vi "Handle Errors.vi"(8 "error in (no error)":errorcluster, 10 "Location":string, 11 "Mock Error Handler In":refnum<class "Mock Error Handler.lvclass">) -> (0 "error out":errorcluster, 3 "Mock Error Handler Out":refnum<class "Mock Error Handler.lvclass">)   [LabVIEW 2020, in "Mock Error Handler.lvclass"]
uses:
  Mock Error Handler.lvclass
  C:/Users/anton/Documents/GitHub/Triarc-Framework/source/Framework/Process/Process.lvclass
  Private/Error Message Data.ctl
  Framework/Process/Process.lvclass/Process.ctl
  <vilib>/AdvancedString/1D String Array to Delimited String.vi
  Framework/Process/Process.lvclass
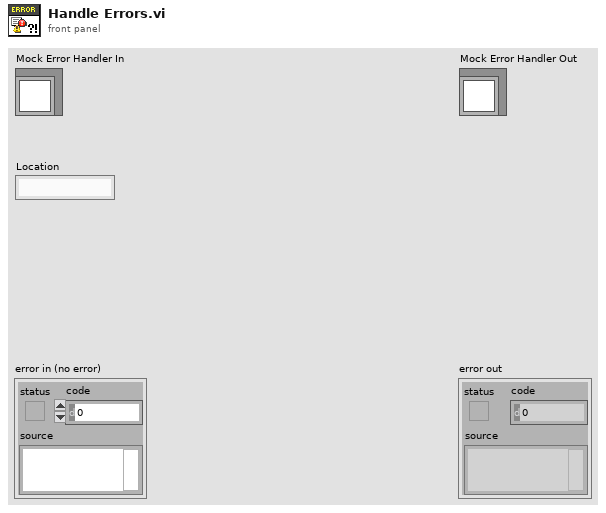
[diagram p1: front panel]
types:
  T1 = typedef "Mock Error Handler.lvclass/Error Message Data.ctl" = cluster{"Error Type":string, "Location":string, "Error":errorcluster}
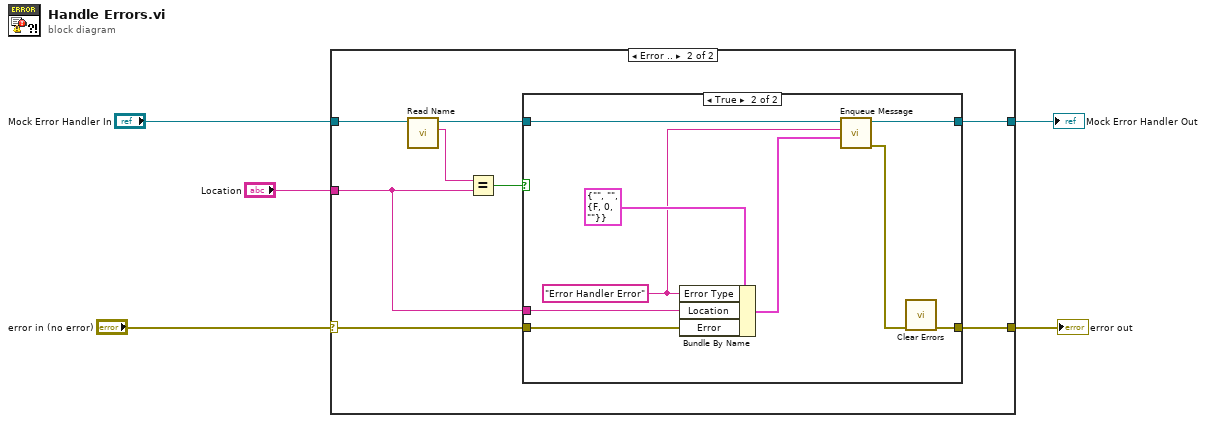
[diagram p0: block diagram]
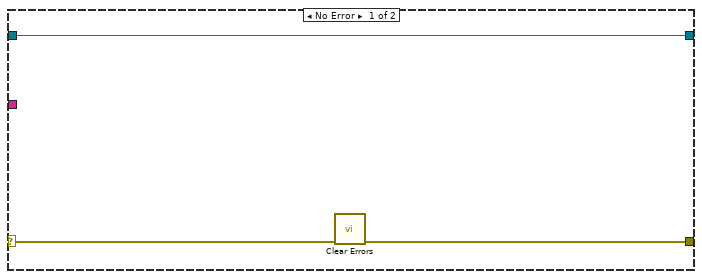
[diagram p2: hidden frame]
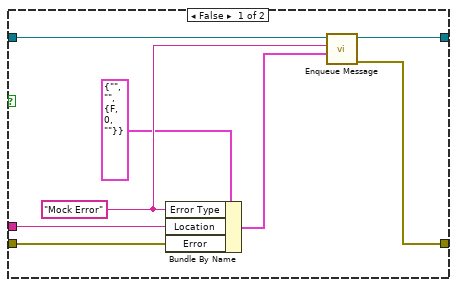
[diagram p3: hidden frame]
diagram:
  n1 = case shown="Error .." "error in (no error)" {
    selector: "error in (no error)" -> [w8 w16]
    tunnel: "Mock Error Handler In" -> [w7 w15]
    tunnel: [w7 w13] -> w5
    tunnel: [w6 w10] -> w1
    tunnel: "Location" -> [_ w11]
    frame No Error {
      n2 = call <vilib>:"Clear Errors.vi"("error in (no error)"=w8) -> ("error out"=w6:errorcluster)  [unwired: 5 in, 1 out]
    }
    frame Error {
      n3 = call-dynamic "Read Name.vi"("Process In"=w15) -> ("Qualified Name"=w12:string, "Process Out"=w14:refnum<class "Mock Error Handler.lvclass">)  [unwired: 7 in, 2 out]
      n4 = Equal?(x=w12, y=w11) -> (x = y?=w9:bool)
      n5 = case shown="True" w9 {
        tunnel: w16 -> [w24 w32]
        tunnel: w14 -> [w23 w31]
        tunnel: [w22 w30] -> w13
        tunnel: w11 -> [w21 w29]
        tunnel: [w18 w25] -> w10
        frame False {
          w19 = "Mock Error" ("Error Type")
          n6 = Bundle By Name(cluster=T1 {"Error Type"="", "Location"="", "Error"={"status"=FALSE, "code"=0, "source"=""}} ("Error Message Data"), "Error Type"=w19, "Location"=w21, "Error"=w24) -> (w20:T1)
          n7 = call "Enqueue Message.vi"("Message Data"=w20, "Message"=w19, "Process In"=w23) -> ("error out"=w18:errorcluster, "Process Out"=w22:refnum<class "Mock Error Handler.lvclass">)  [unwired: 7 in]
        }
        frame True {
          w27 = "Error Handler Error" ("Error Type")
          n8 = Bundle By Name(cluster=T1 {"Error Type"="", "Location"="", "Error"={"status"=FALSE, "code"=0, "source"=""}} ("Error Message Data"), "Error Type"=w27, "Location"=w29, "Error"=w32) -> (w28:T1)
          n9 = call "Enqueue Message.vi"("Message Data"=w28, "Message"=w27, "Process In"=w31) -> ("error out"=w26:errorcluster, "Process Out"=w30:refnum<class "Mock Error Handler.lvclass">)  [unwired: 7 in]
          n10 = call <vilib>:"Clear Errors.vi"("error in (no error)"=w26) -> ("error out"=w25:errorcluster)  [unwired: 5 in, 1 out]
        }
      }
    }
  }
  "error out" <- w1
  "Mock Error Handler Out" <- w5
